vi "L5K Global.vi"() -> ()   [LabVIEW 2010]
panel:
  in  "Ring":i16(ring) items=["Unchanged"=-1, "Online"=0, "Loaded"=1, "Inspecting"=2, "Ready"=3, "Busy"=4, "Acquiring"=5, "Acquisition Done"=6, "Error"=7]
  in  "Numeric 2":dbl
  in  "Numeric":dbl
  in  "Input Register":cluster{}
  in  "Reserved Address Space":dbl
  in  "Output Assembly Size":dbl
  in  "Output Assembly Instance":dbl
  in  "Input Assembly Size":dbl
  in  "Input Assembly Instance":dbl
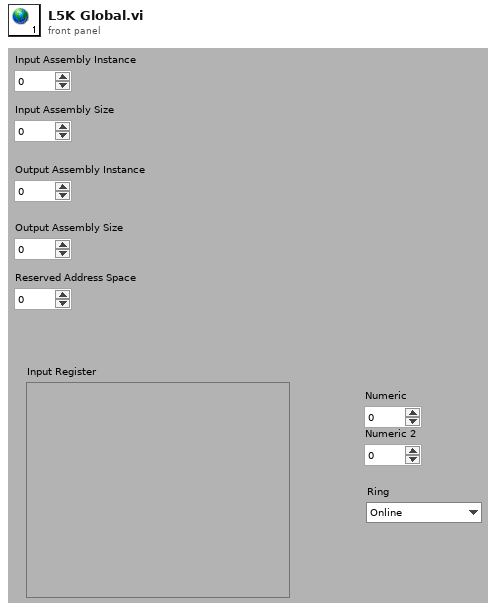
[diagram p1: front panel]
diagram:
